vi "Write to PIC Board.vi"(5 "Read after write":bool=TRUE, 7 "Delay between writes":u32, 8 "error in (no error)":errorcluster, 9 "Ignore address in return":bool, 10 "String to write":string, 11 "VISA Refnum in":refnum<visa-resource-name>) -> (0 "Error Out":errorcluster, 2 "Return":string[](array[string]))   [LabVIEW 2020, in "PIC-Device.lvclass"]
doc: "SubVI wating on the PIC board to respond. It reads the respond and trims it"
uses:
  PIC-Device.lvclass
  <vilib>/Instr/_visa.llb/Select Event Type.ctl
  <vilib>/Utility/error.llb/whitespace.ctl
panel:
  out "Return":string
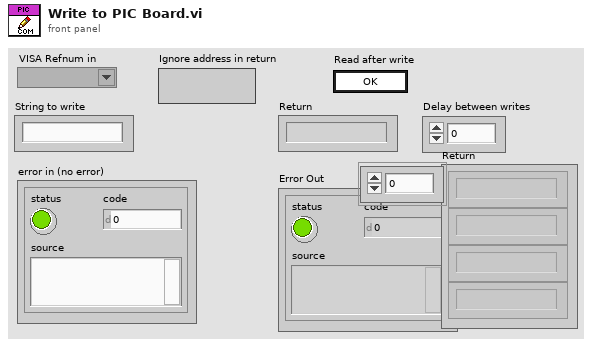
[diagram p1: front panel]
types:
  T1 = typedef "whitespace.ctl" = u16
  T2 = typedef "Select Event Type.ctl" = u32
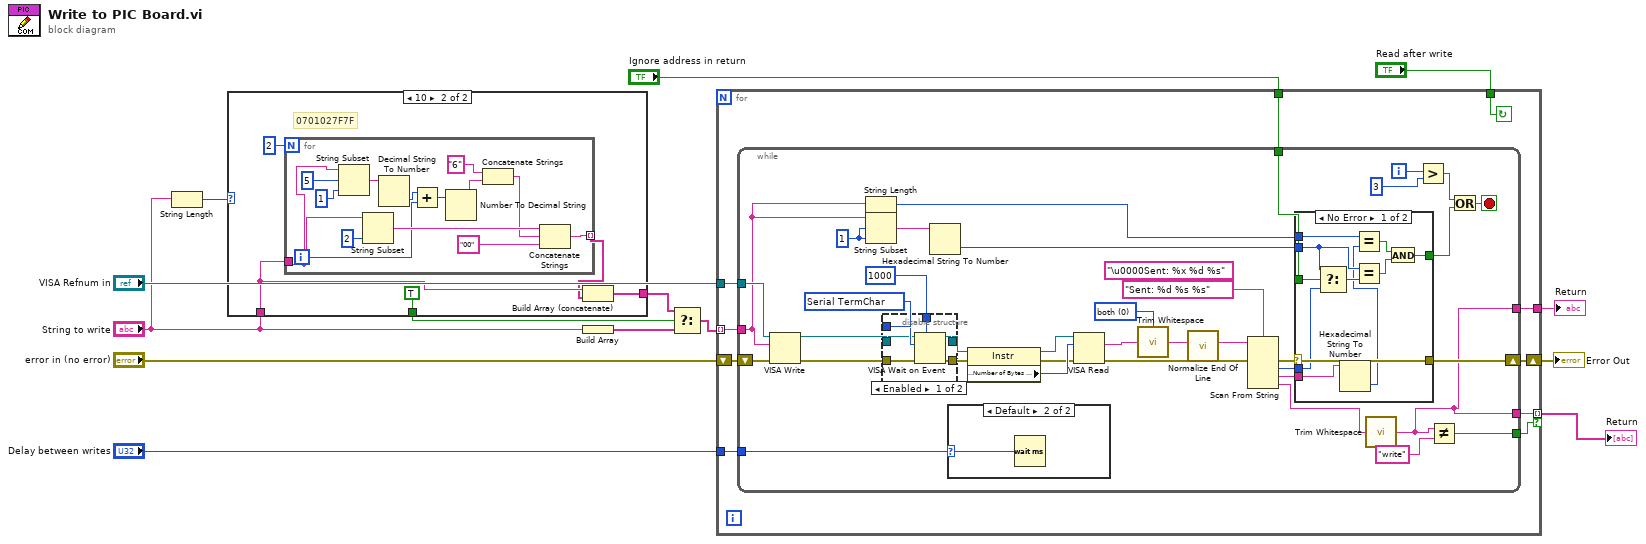
[diagram p0: block diagram]
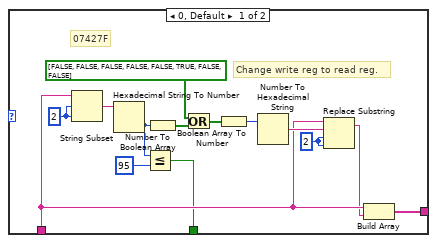
[diagram p2: hidden frame]
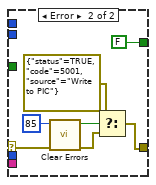
[diagram p5: hidden frame]
diagram:
  n1 = String Length(string="String to write") -> (length=w2:i32)
  n2 = case shown="10" w2 {
    tunnel: "String to write" -> [w18 w32]
    tunnel: [w17 w33] -> w9
    tunnel: [w16 TRUE] -> w8
    frame 0, Default {
      w22 = 2 ("offset (0)")
      w21 = 2 ("length (rest)")
      # "07427F"
      # "Change write reg to read reg."
      n3 = String Subset(string=w18, offset (0)=w21, length (rest)=w21) -> (substring=w24:string)
      n4 = Hexadecimal String To Number(string=w24) -> (number=w20:u32)  [unwired: 2 in, 1 out]
      n5 = Less Or Equal?(x=w20, y=u32 95) -> (x <= y?=w16:bool)
      n6 = Number To Boolean Array(number=w20) -> (Boolean array=w27:bool[])
      n7 = Or(x=bool[] [FALSE, FALSE, FALSE, FALSE, FALSE, TRUE, FALSE, FALSE] ("Boolean array"), y=w27) -> (x .or. y?=w26:bool[])
      n8 = Boolean Array To Number(Boolean array=w26) -> (number=w25:u32)
      n9 = Number To Hexadecimal String(2:w25) -> (0:w23:string)  [unwired: 1 in]
      n10 = Replace Substring(2:w22, 3:w22, 4:w23, 5:w18) -> (1:w15:string)  [unwired: 1 out]
      n11 = Build Array(w18, w15) -> (w17:string[])
    }
    frame 10 {
      # "0701027F7F"
      n12 = for {
        N: 2 -> [_]
        tunnel: w32 -> [w45]
        tunnel: [w40] -> w31 mode=indexing
        i -> [w34]
        n13 = String Subset(string=w45, offset (0)=5, length (rest)=1 ("length (rest)")) -> (substring=w35:string)
        n14 = String Subset(string=w45, length (rest)=2 ("length (rest)")) -> (substring=w42:string)  [unwired: 1 in]
        n15 = Decimal String To Number(string=w35) -> (number=w38:i32)  [unwired: 2 in, 1 out]
        n16 = Add(x=w38, y=w34) -> (x+y=w37:i32)
        n17 = Number To Decimal String(number=w37) -> (decimal integer string=w36:string)  [unwired: 1 in]
        n18 = Concatenate Strings("6" ("string"), w36) -> (w39:string)
        n19 = Concatenate Strings(w42, w39, "00" ("String to write")) -> (w40:string)
      }
      n20 = Build Array (concatenate)(w32, w31) -> (w33:string[])
    }
  }
  n21 = Build Array("String to write") -> (w10:string[])
  n22 = Select(t=w9, s=w8, f=w10) -> (s? t:f=w7:string[])
  n23 = for {
    tunnel: "VISA Refnum in" -> [w56]
    tunnel: [w54] -> w11
    shift-right: [w55] -> w12
    shift-left: "error in (no error)" -> [w57]
    tunnel: w7 -> [w53] mode=indexing
    tunnel: "Delay between writes" -> [w52]
    tunnel: "Ignore address in return" -> [w51]
    tunnel: "Read after write" -> [w50]
    tunnel: [w49] -> w1 mode=indexing if=w48
    stop <- w50 continue-if-true
    n24 = while {
      tunnel: w53 -> [w81]
      tunnel: w56 -> [w84]
      shift-right: [w73] -> w55
      shift-left: w57 -> [w85]
      tunnel: [w60] -> w54
      tunnel: w52 -> [w63]
      tunnel: w51 -> [w62]
      tunnel: [w60] -> w49
      tunnel: [w58] -> w48
      i -> [w72]
      stop <- w70 stop-if-true
      (unwired) "\u0000Sent: %x %d %s" ("format string")
      w64 = 1 ("length (rest)")
      w86 = T1 0 items=["both", "start of string", "end of string"] ("location (both)")
      w89 = T2 1073684516 items=["Service Request"=1073684491, "Trigger"=3221168138, "Clear"=1073684493, "VXI Signal"=1073684512, "VXI/VME Interrupt"=3221168161, "VXI/VME Sysfail"=1073684509, "VXI/VME Sysreset"=1073684510, "GPIB CIC"=1073684498, "GPIB Talk"=1073684499, "GPIB Listen"=1073684500, "PXI Interrupt"=1073684514, "Serial Break"=1073684515, "Serial TermChar"=1073684516, "Serial CTS"=1073684521, "Serial DSR"=1073684522, "Serial DCD"=1073684524, "Serial RI"=1073684526, "Serial Character"=1073684533, "USB Interrupt"=1073684535, "All Enabled"=1073709055] ("Event Type")
      n25 = VISA Write(VISA resource name=w84, write buffer=w81, error in (no error)=w85) -> (VISA resource name out=w83:refnum<visa-resource-name>, error out=w82:errorcluster)  [unwired: 1 out]
      n26 = String Length(string=w81) -> (length=w75:i32)
      n27 = String Subset(string=w81, offset (0)=w64, length (rest)=w64) -> (substring=w80:string)
      n28 = disable-structure shown="Enabled" {
        disable-tunnel: [w101 w102] -> w91
        disable-tunnel: [w100 w103] -> w90
        disable-tunnel: w89 -> [w99 _]
        disable-tunnel: u32 1000 ("timeout (0)") -> [w98 _]
        disable-tunnel: w83 -> [w97 w103]
        disable-tunnel: w82 -> [w96 w102]
        frame Enabled {
          n29 = VISA Wait on Event(7:w98, 8:w96, 10:w99, 11:w97) -> (0:w101:errorcluster, 3:w100:refnum<visa-resource-name>)  [unwired: 1 in, 2 out]
        }
        frame Disabled {
        }
      }
      n30 = Hexadecimal String To Number(string=w80) -> (number=w74:u32)  [unwired: 2 in, 1 out]
      n31 = case shown="Default" w63 {
        selector: w63 -> [_ w95]
        frame 0 {
        }
        frame Default {
          n32 = Wait (ms)(milliseconds to wait=w95) -> ()  [unwired: 1 out]
        }
      }
      n33 = property class="Instr"(reference=w90, error in=w91) -> (reference out=w92:refnum<visa-resource-name>, error out=w93:errorcluster, "Serial Settings:Number of Bytes at Serial Port"=w94:u32)
      n34 = VISA Read(VISA resource name=w92, byte count=w94, error in (no error)=w93) -> (read buffer=w87:string, error out=w79:errorcluster)  [unwired: 2 out]
      n35 = call <vilib>:"Trim Whitespace.vi"("string"=w87, "location (both)"=w86) -> ("trimmed string"=w66:string)
      n36 = call <vilib>:"Normalize End Of Line.vi"("string in"=w66) -> ("string out"=w65:string)  [unwired: 7 in]
      n37 = Scan From String(format string="Sent: %d %s %s", input string=w65, error in=w79) -> (error out=w78:errorcluster, output 1=w77:i32, output 2=w76:string, output 3=w61:string)  [unwired: 4 in, 2 out]
      n38 = case shown="No Error" w78 {
        selector: w78 -> [w110 w121]
        tunnel: w77 -> [w108 _]
        tunnel: w76 -> [w105 _]
        tunnel: w75 -> [w114 _]
        tunnel: w74 -> [w107 _]
        tunnel: [w111 FALSE] -> w68
        tunnel: [w110 w116] -> w73
        tunnel: w62 -> [w109 _]
        frame No Error {
          n39 = Select(t=w107, s=w109, f=w108) -> (s? t:f=w106:u32)
          n40 = Hexadecimal String To Number(string=w105) -> (number=w104:u32)  [unwired: 2 in, 1 out]
          n41 = Equal?(x=w114, y=w104) -> (x = y?=w113:bool)
          n42 = Equal?(x=w107, y=w106) -> (x = y?=w112:bool)
          n43 = And(x=w113, y=w112) -> (x .and. y?=w111:bool)
        }
        frame Error {
          n44 = call <vilib>:"Clear Errors.vi"("error in (no error)"=w121, "specific error code to clear (0: all)"=85) -> ("error out"=w117:errorcluster, "specific error cleared?"=w118:bool)  [unwired: 4 in]
          n45 = Select(t=errorcluster {"status"=TRUE, "code"=5001, "source"="Write to PIC"}, s=w118, f=w117) -> (s? t:f=w116:errorcluster)
        }
      }
      n46 = call <vilib>:"Trim Whitespace.vi"("string"=w61) -> ("trimmed string"=w60:string)  [unwired: 1 in]
      n47 = Greater?(x=w72, y=3) -> (0:w69:bool)
      n48 = Not Equal?(x=w60, y="write") -> (x != y?=w58:bool)
      n49 = Or(x=w69, y=w68) -> (x .or. y?=w70:bool)
    }
  }
  "Error Out" <- w12
  "Return" <- w11
  "Return" <- w1
